vi "KB-二维数组算差值.vi"(11 "子数组":dbl[][](array[numeric])) -> (3 "差值":dbl)   [LabVIEW 2015]
uses:
  <vilib>/Math Plots/3D Math Plots/3D Surface/3D Surface XCtrl/3D Surface.xctl
  <vilib>/Math Plots/3D Math Plots/3D Surface/3D Surface Datatype/Public/Plot Helper (Matrix).vi
  <vilib>/Math Plots/3D Math Plots/3D Surface/3D Surface Datatype/3D Surface Datatype.lvclass
  <vilib>/Analysis/NI_AAL_SigProc.lvlib
panel:
  out "已排序的数组":dbl[](array[numeric])
  out "x-1":i32
  out "元素 2":dbl
  out "元素":dbl
  out "数值":dbl
  out "最大值":dbl
  out "数组":dbl[](array[numeric])
  out "# found":i32 caption="找到个数"
  out "Locations":dbl[](array[numeric]) caption="位置"
  out "波形图":dbl[](graph)
  out "3D Surface 2":refnum<class "3D Plot Datatype.lvclass">[](xcontrol) caption="三维曲面"
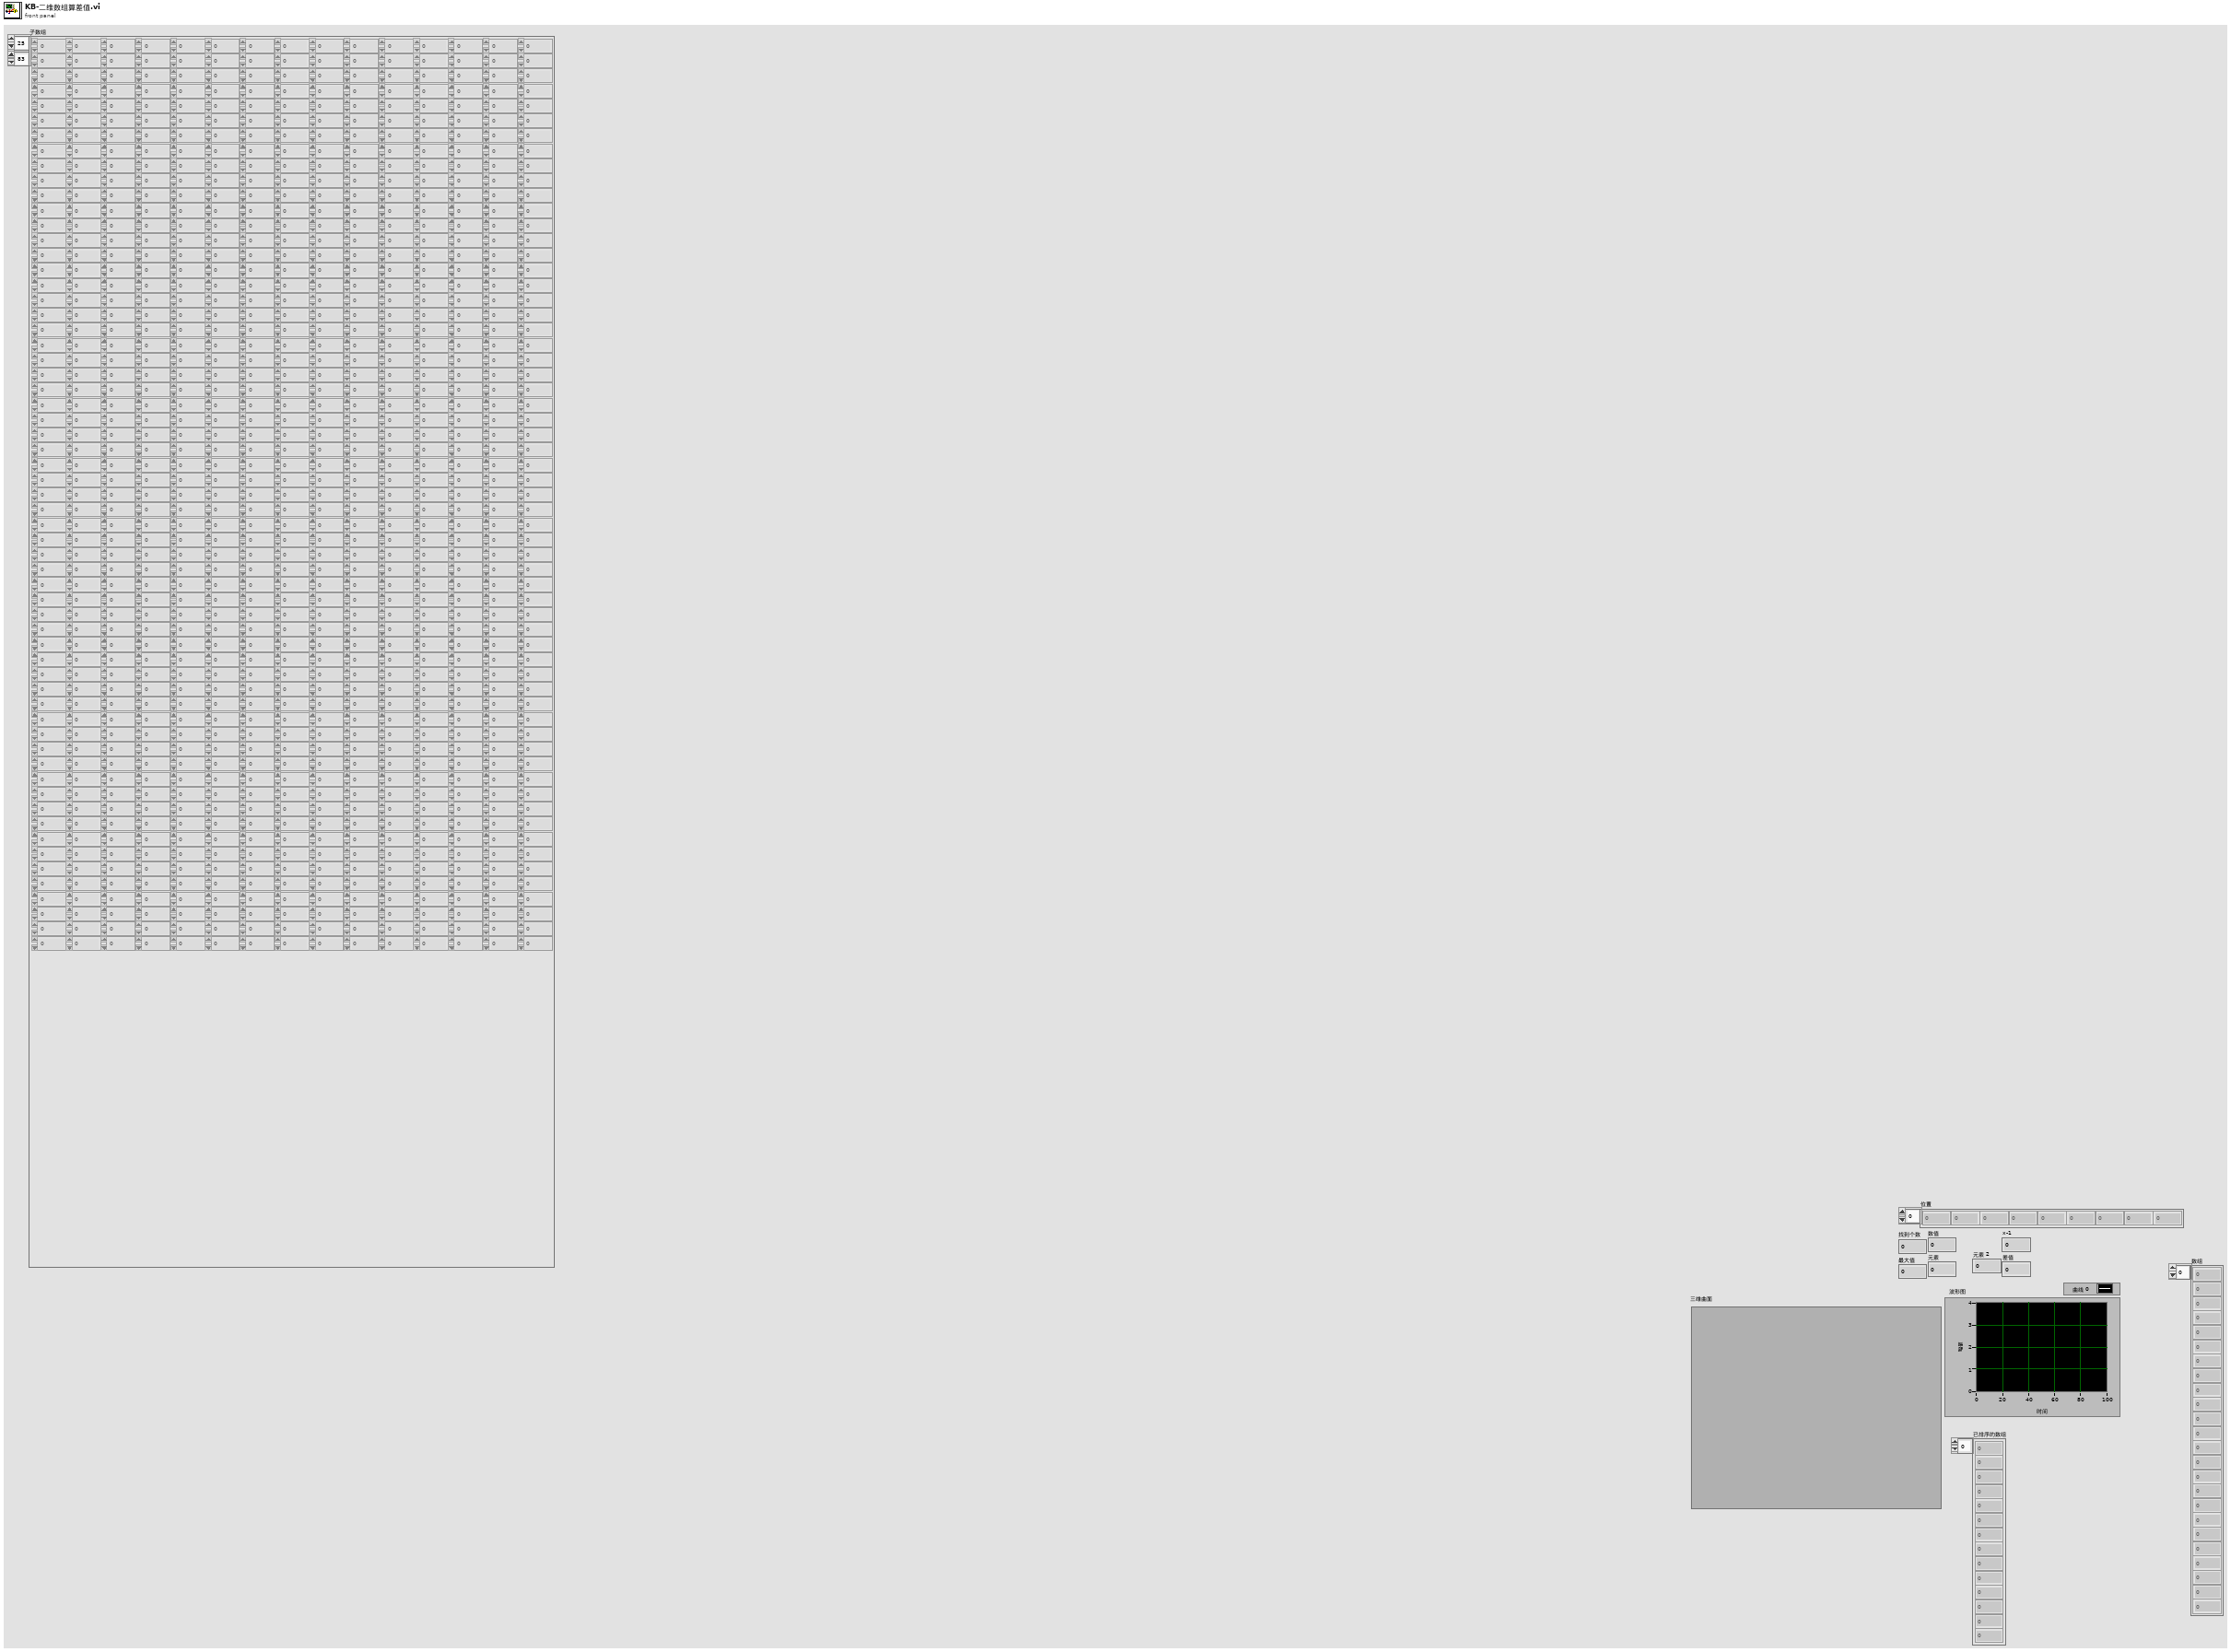
[diagram p1: front panel]
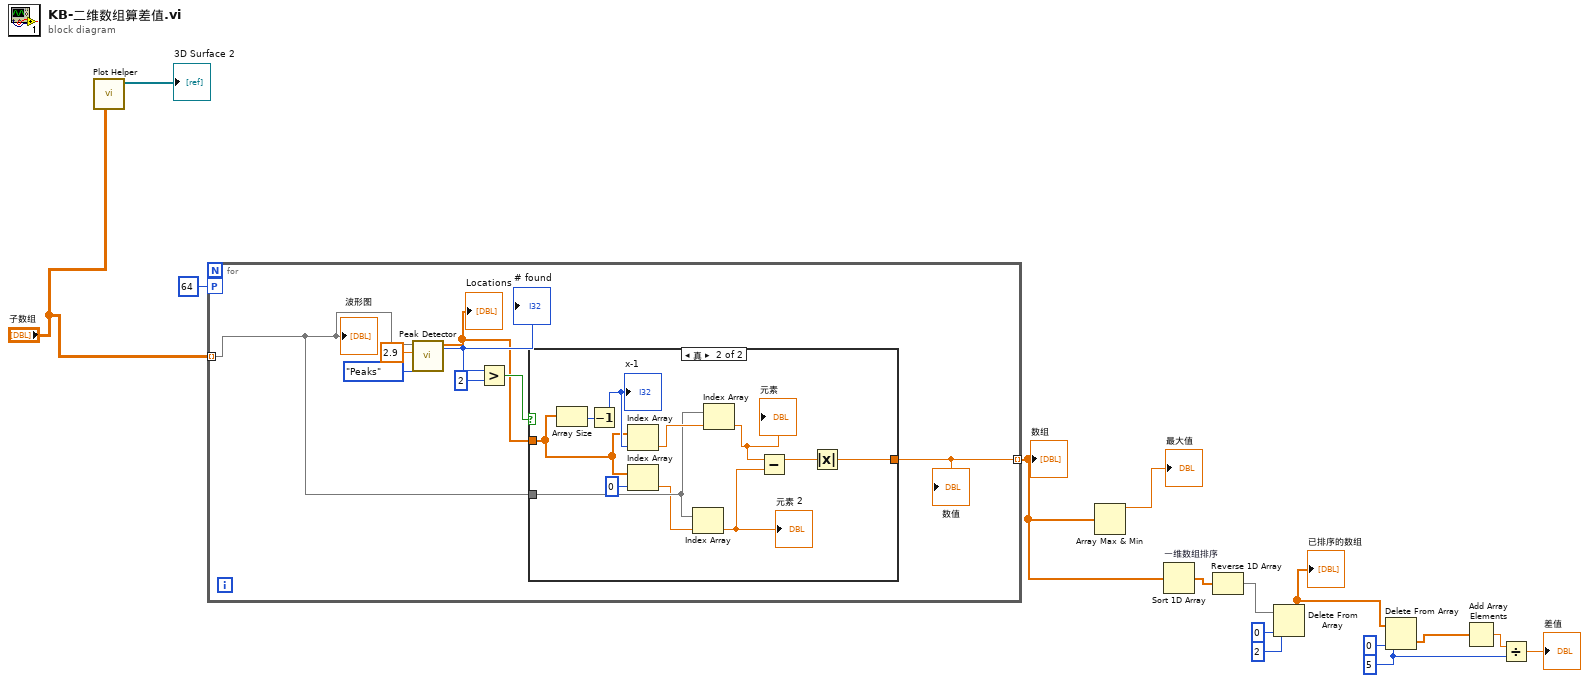
[diagram p0: block diagram]
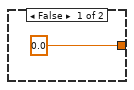
[diagram p2: hidden frame]
diagram:
  w3 = 5 ("长度")
  n1 = call-poly <vilib>:"Plot Helper.vi"("z matrix"="子数组") -> ("3D Plot lvclass Array out"=→"3D Surface 2":refnum<class "3D Plot Datatype.lvclass">[])  [unwired: 5 in, 5 out]
  n2 = for {
    tunnel: "子数组" -> [w17] mode=indexing
    tunnel: [w16] -> w12 mode=indexing
    workers-P: 64 -> [_]
    n3 = call <vilib>:"Peak Detector.vi"("peaks/valleys"=enum32{"Peaks", "Valleys"}."Peaks", "threshold"=2.9, "X"=w17) -> ("Locations"=w18:dbl[], "# found"=w21:i32)  [unwired: 4 in, 3 out]
    "Locations" <- w18
    "# found" <- w21
    n4 = Greater?(x=w21, y=2) -> (0:w19:bool)
    n5 = case shown="真" w19 {
      tunnel: w18 -> [_ w30]
      tunnel: w17 -> [_ w28]
      tunnel: [0.0 w31] -> w16
      frame False {
      }
      frame True {
        n6 = Array Size(array=w30) -> (size(s)=w35:i32)
        n7 = Decrement(x=w35) -> (x-1=w34:i32)
        "x-1" <- w34
        n8 = Index Array(array=w30, index=w34) -> (element=w29:dbl)
        n9 = Index Array(array=w30, index=0 ("索引")) -> (element=w27:dbl)
        n10 = Index Array(array=w28, index=w27) -> (element=w25:dbl)
        "元素 2" <- w25
        n11 = Index Array(array=w28, index=w29) -> (element=w26:dbl)
        "元素" <- w26
        n12 = Subtract(x=w26, y=w25) -> (x-y=w32:dbl)
        n13 = Absolute Value(x=w32) -> (abs(x)=w31:dbl)
      }
    }
    "数值" <- w16
    "波形图" <- w17
  }
  "数组" <- w12
  n14 = Array Max & Min(array=w12) -> (max value=→"最大值":dbl)  [unwired: 3 out]
  n15 = Sort 1D Array "一维数组排序"(array=w12) -> (sorted array=w11:dbl[])
  n16 = Reverse 1D Array(array=w11) -> (reversed array=w8:dbl[])
  n17 = Delete From Array(array=w8, length=2 ("长度"), index=0 ("索引")) -> (array with subset deleted=w7:dbl[])  [unwired: 1 out]
  "已排序的数组" <- w7
  n18 = Delete From Array(array=w7, length=w3, index=0 ("索引")) -> (deleted portion=w5:dbl[])  [unwired: 1 out]
  n19 = Add Array Elements(numeric array=w5) -> (sum=w4:dbl)
  n20 = Divide(x=w4, y=w3) -> (x/y=→"差值":dbl)
